vi "conv EOL.vi"(10 "standard output in":string) -> (2 "result string":string)   [LabVIEW 2020, in "Approval Tests.lvlib"]
uses:
  Approval Tests.lvlib
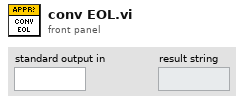
[diagram p1: front panel]
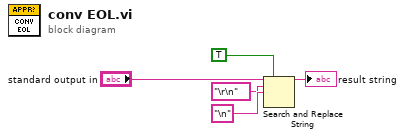
[diagram p0: block diagram]
diagram:
  n1 = Search and Replace String(replace all?=TRUE ("replace all? (F)"), input string="standard output in", search string="\r\n", replace string="\n") -> (result string=→"result string":string)  [unwired: 4 in, 3 out]
